vi "Conversion.vi"() -> ()   [LabVIEW 2014]
doc: "This is the easiest way to capture a frame from a camera."
uses:
  MSC Image_class/controls/Image Type.ctl
  MSC Image_class/MSC Image.lvclass
panel:
  out "error out":errorcluster
  out "picture":picture
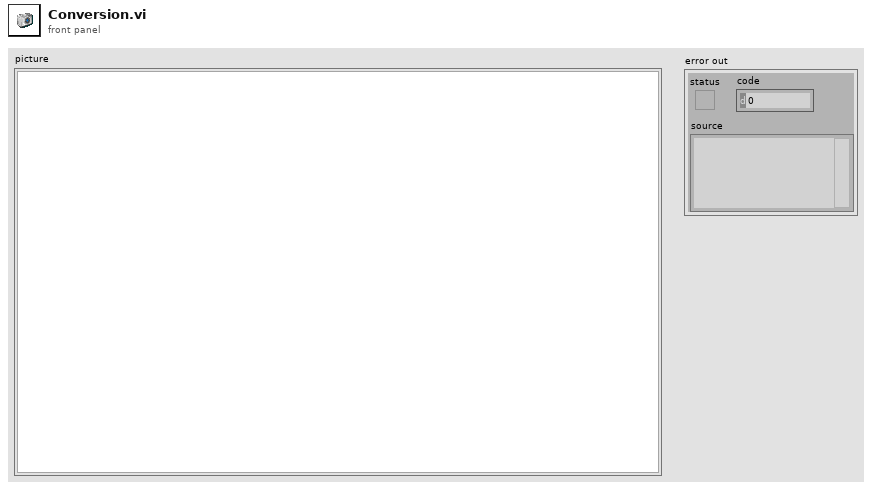
[diagram p1: front panel]
types:
  T1 = typedef "MSC Image.lvclass/Image Type.ctl" = i32
  T2 = typedef "imagedata.ctl" = cluster{"image type":i32, "image depth":i32, "image":u8[], "mask":u8[], "colors":u32[], "Rectangle":cluster{"left":i16, "top":i16, "right":i16, "bottom":i16}}
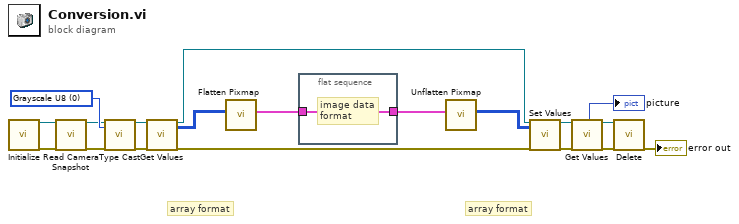
[diagram p0: block diagram]
diagram:
  w16 = T1 0 items=["Grayscale U8"=0, "Grayscale U16"=2, "Grayscale Single"=5, "Grayscale Double"=6, "RGB U8"=16] ("Image Type")
  # "array format"
  # "array format"
  n1 = call "Initialize.vi"() -> ("image out"=w19:refnum<class "MSC Image.lvclass">, "error out"=w18:errorcluster)  [unwired: 18 in]
  n2 = call-dynamic "Read Camera Snapshot.vi"("image in"=w19, "error in (no error)"=w18) -> ("image out"=w15:refnum<class "MSC Image.lvclass">, "error out"=w8:errorcluster)  [unwired: 16 in]
  n3 = call-dynamic "Type Cast.vi"("image in"=w15, "Image Type"=w16, "error in (no error)"=w8) -> ("image out"=w14:refnum<class "MSC Image.lvclass">, "error out"=w7:errorcluster)  [unwired: 15 in]
  n4 = call-dynamic "Get Values.vi"("image in"=w14, "error in (no error)"=w7) -> ("image out"=w11:refnum<class "MSC Image.lvclass">, "imageData U8"=w13:u8[][], "error out"=w6:errorcluster)  [unwired: 10 in, 5 out]
  n5 = call <vilib>:"Flatten Pixmap.vi"("8-bit pixmap"=w13) -> ("image data"=w10:T2)  [unwired: 10 in]
  n6 = flat-sequence {
    tunnel: w10 -> [w20]
    tunnel: [w20] -> w9
    frame #0 {
      # "image data\nformat"
    }
  }
  n7 = call <vilib>:"Unflatten Pixmap.vi"("image data"=w9) -> ("8-bit pixmap"=w12:u8[][])  [unwired: 4 in, 6 out]
  n8 = call-dynamic "Set Values.vi"("image in"=w11, "imageData U8"=w12, "error in (no error)"=w6) -> ("image out"=w5:refnum<class "MSC Image.lvclass">, "error out"=w2:errorcluster)  [unwired: 15 in]
  n9 = call-dynamic "Get Values.vi"("image in"=w5, "error in (no error)"=w2) -> ("picture"=→"picture":picture, "image out"=w4:refnum<class "MSC Image.lvclass">, "error out"=w1:errorcluster)  [unwired: 10 in, 5 out]
  n10 = call-dynamic "Delete.vi"("image in"=w4, "error in (no error)"=w1) -> ("error out"=→"error out":errorcluster)  [unwired: 17 in]
